vi "Drive Test.vi"   [LabVIEW 2018]
types:
  T1 = cluster{"Reverse (T) / Normal (F)":bool, "Power Scaling (1=Normal) ":dbl, "Deadband Value":dbl}
  T2 = typedef "WPI_MotorControlDeviceRef.ctl" = cluster{"DeviceStatus":errorcluster, "Type":T3, "PWM":cluster{"PWM Channel":T4, "DeadBand":T5}, "CAN":cluster{"Device Number":u8, "SetOutput VI Ref":variant, "GetOutput VI Ref":variant, "Enable VI Ref":variant, "Disable VI Ref":variant, "Data":variant}, "Invert":bool, "DIO PWM":cluster{"PWM \"Enable\" Channel":T4, "DIOChannel":T6, "PWM Rate":dbl}}
  T3 = typedef "WPI_MotorControlType.ctl" = enum16{"PWM", "CAN", "DIO PWM"}
  T4 = typedef "FPGA_DIOPWMChannel.ctl" = enum8{"PWM 0", "PWM 1", "PWM 2", "PWM 3", "PWM 4", "PWM 5", "PWM 6", "PWM 7", "PWM 8", "PWM 9", "PWM MXP 0", "PWM MXP 1", "PWM MXP 2", "PWM MXP 3", "PWM MXP 4", "PWM MXP 5", "PWM MXP 6", "PWM MXP 7", "PWM MXP 8", "PWM MXP 9", "Invalid"}
  T5 = typedef "WPI_PWMDeadband.ctl" = cluster{"Name":string, "maxPositivePwm":i32, "minPositivePwm":i32, "centerPwm":i32, "maxNegativePwm":i32, "minNegativePwm":i32, "angularRange":u16}
  T6 = typedef "FPGA_DIOChannel.ctl" = enum8{"DIO 0", "DIO 1", "DIO 2", "DIO 3", "DIO 4", "DIO 5", "DIO 6", "DIO 7", "DIO 8", "DIO 9", "DIO MXP 0", "DIO MXP 1", "DIO MXP 2", "DIO MXP 3", "DIO MXP 4", "DIO MXP 5", "DIO MXP 6", "DIO MXP 7", "DIO MXP 8", "DIO MXP 9", "DIO MXP 10", "DIO MXP 11", "DIO MXP 12", "DIO MXP 13", "DIO MXP 14", "DIO MXP 15", "SPI Port CS1", "SPI Port CS2", "SPI Port CS3", "SPI Port MISO", "SPI Port MOSI", "Invalid"}
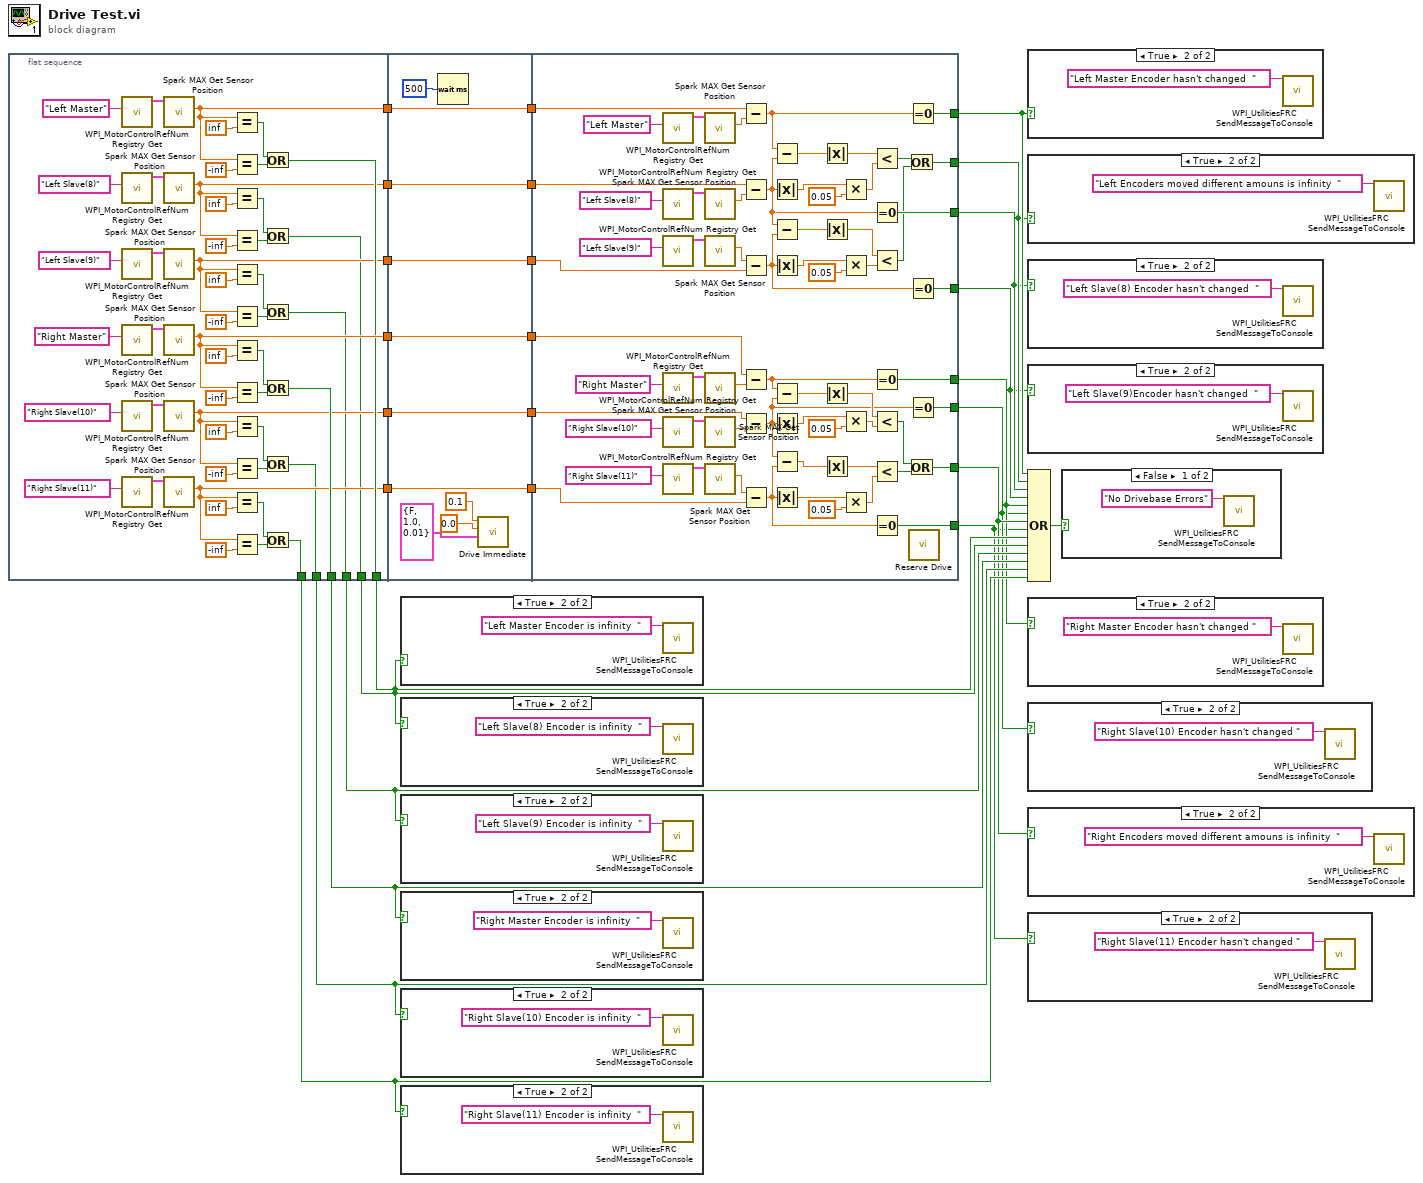
[diagram p0: block diagram]
diagram:
  n1 = flat-sequence {
    tunnel: [w63] -> w27
    tunnel: [w62] -> w26
    tunnel: [w61] -> w14
    tunnel: [w60] -> w11
    tunnel: [w47] -> w22
    tunnel: [w46] -> w20
    tunnel: [w44] -> w17
    tunnel: [w45] -> w16
    tunnel: [w31] -> w13
    tunnel: [w30] -> w12
    tunnel: [w29] -> w10
    tunnel: [w28] -> w9
    tunnel: w27 -> [w82]
    tunnel: [w82] -> w25
    tunnel: w26 -> [w81]
    tunnel: [w81] -> w24
    tunnel: [w79] -> w23
    tunnel: w22 -> [w79]
    tunnel: [w78] -> w21
    tunnel: w20 -> [w78]
    tunnel: [w76] -> w19
    tunnel: [w77] -> w18
    tunnel: w17 -> [w76]
    tunnel: w16 -> [w77]
    tunnel: w25 -> [w143]
    tunnel: w24 -> [w128]
    tunnel: [w133] -> w8
    tunnel: [w126] -> w3
    tunnel: w23 -> [w130]
    tunnel: w21 -> [w90]
    tunnel: w19 -> [w125]
    tunnel: w18 -> [w92]
    tunnel: [w132] -> w6
    tunnel: [w129] -> w4
    tunnel: [w123] -> w2
    tunnel: [w122] -> w1
    tunnel: [w88] -> w7
    tunnel: [w87] -> w5
    frame #0 {
      n2 = call <vilib>:"WPI_MotorControlRefNum Registry Get.vi"("refnum name"="Left Master") -> ("MotorControlDevRef"=w75:T2)  [unwired: 9 in, 1 out]
      n3 = call <vilib>:"WPI_MotorControlRefNum Registry Get.vi"("refnum name"="Left Slave(8)") -> ("MotorControlDevRef"=w49:T2)  [unwired: 9 in, 1 out]
      n4 = call <vilib>:"WPI_MotorControlRefNum Registry Get.vi"("refnum name"="Left Slave(9)") -> ("MotorControlDevRef"=w48:T2)  [unwired: 9 in, 1 out]
      n5 = call <vilib>:"WPI_MotorControlRefNum Registry Get.vi"("refnum name"="Right Master") -> ("MotorControlDevRef"=w74:T2)  [unwired: 9 in, 1 out]
      n6 = call <vilib>:"WPI_MotorControlRefNum Registry Get.vi"("refnum name"="Right Slave(10)") -> ("MotorControlDevRef"=w42:T2)  [unwired: 9 in, 1 out]
      n7 = call <vilib>:"WPI_MotorControlRefNum Registry Get.vi"("refnum name"="Right Slave(11)") -> ("MotorControlDevRef"=w43:T2)  [unwired: 9 in, 1 out]
      n8 = call <vilib>:"Spark MAX Get Sensor Position.vi"("MotorControlDevRef in"=w75) -> ("Sensor Position"=w63:dbl)  [unwired: 7 in, 3 out]
      n9 = call <vilib>:"Spark MAX Get Sensor Position.vi"("MotorControlDevRef in"=w49) -> ("Sensor Position"=w47:dbl)  [unwired: 7 in, 3 out]
      n10 = call <vilib>:"Spark MAX Get Sensor Position.vi"("MotorControlDevRef in"=w48) -> ("Sensor Position"=w46:dbl)  [unwired: 7 in, 3 out]
      n11 = call <vilib>:"Spark MAX Get Sensor Position.vi"("MotorControlDevRef in"=w74) -> ("Sensor Position"=w62:dbl)  [unwired: 7 in, 3 out]
      n12 = call <vilib>:"Spark MAX Get Sensor Position.vi"("MotorControlDevRef in"=w42) -> ("Sensor Position"=w44:dbl)  [unwired: 7 in, 3 out]
      n13 = call <vilib>:"Spark MAX Get Sensor Position.vi"("MotorControlDevRef in"=w43) -> ("Sensor Position"=w45:dbl)  [unwired: 7 in, 3 out]
      n14 = Equal?(x=w63, y=inf) -> (x = y?=w68:bool)
      n15 = Equal?(x=w63, y=-inf) -> (x = y?=w69:bool)
      n16 = Equal?(x=w47, y=inf) -> (x = y?=w56:bool)
      n17 = Equal?(x=w47, y=-inf) -> (x = y?=w57:bool)
      n18 = Equal?(x=w46, y=inf) -> (x = y?=w55:bool)
      n19 = Equal?(x=w46, y=-inf) -> (x = y?=w54:bool)
      n20 = Equal?(x=w62, y=inf) -> (x = y?=w67:bool)
      n21 = Equal?(x=w62, y=-inf) -> (x = y?=w66:bool)
      n22 = Equal?(x=w44, y=inf) -> (x = y?=w35:bool)
      n23 = Equal?(x=w44, y=-inf) -> (x = y?=w34:bool)
      n24 = Equal?(x=w45, y=inf) -> (x = y?=w36:bool)
      n25 = Equal?(x=w45, y=-inf) -> (x = y?=w37:bool)
      n26 = Or(x=w68, y=w69) -> (x .or. y?=w61:bool)
      n27 = Or(x=w56, y=w57) -> (x .or. y?=w31:bool)
      n28 = Or(x=w55, y=w54) -> (x .or. y?=w30:bool)
      n29 = Or(x=w67, y=w66) -> (x .or. y?=w60:bool)
      n30 = Or(x=w35, y=w34) -> (x .or. y?=w29:bool)
      n31 = Or(x=w36, y=w37) -> (x .or. y?=w28:bool)
    }
    frame #1 {
      n32 = Wait (ms)(milliseconds to wait=u32 500) -> ()  [unwired: 1 out]
      n33 = call "Drive Immediate.vi"("Modifiers"=T1 {"Reverse (T) / Normal (F)"=FALSE, "Power Scaling (1=Normal) "=1.0, "Deadband Value"=0.01}, "Right Setpoint (Turning)"=0.0, "Left Setpoint (Power)"=0.1) -> ()  [unwired: 8 in, 1 out]
    }
    frame #2 {
      n34 = call <vilib>:"WPI_MotorControlRefNum Registry Get.vi"("refnum name"="Left Master") -> ("MotorControlDevRef"=w144:T2)  [unwired: 9 in, 1 out]
      n35 = call <vilib>:"WPI_MotorControlRefNum Registry Get.vi"("refnum name"="Left Slave(8)") -> ("MotorControlDevRef"=w140:T2)  [unwired: 9 in, 1 out]
      n36 = call <vilib>:"WPI_MotorControlRefNum Registry Get.vi"("refnum name"="Left Slave(9)") -> ("MotorControlDevRef"=w141:T2)  [unwired: 9 in, 1 out]
      n37 = call <vilib>:"WPI_MotorControlRefNum Registry Get.vi"("refnum name"="Right Master") -> ("MotorControlDevRef"=w145:T2)  [unwired: 9 in, 1 out]
      n38 = call <vilib>:"WPI_MotorControlRefNum Registry Get.vi"("refnum name"="Right Slave(10)") -> ("MotorControlDevRef"=w135:T2)  [unwired: 9 in, 1 out]
      n39 = call <vilib>:"WPI_MotorControlRefNum Registry Get.vi"("refnum name"="Right Slave(11)") -> ("MotorControlDevRef"=w134:T2)  [unwired: 9 in, 1 out]
      n40 = call <vilib>:"Spark MAX Get Sensor Position.vi"("MotorControlDevRef in"=w144) -> ("Sensor Position"=w142:dbl)  [unwired: 7 in, 3 out]
      n41 = call <vilib>:"Spark MAX Get Sensor Position.vi"("MotorControlDevRef in"=w140) -> ("Sensor Position"=w131:dbl)  [unwired: 7 in, 3 out]
      n42 = call <vilib>:"Spark MAX Get Sensor Position.vi"("MotorControlDevRef in"=w141) -> ("Sensor Position"=w91:dbl)  [unwired: 7 in, 3 out]
      n43 = call <vilib>:"Spark MAX Get Sensor Position.vi"("MotorControlDevRef in"=w145) -> ("Sensor Position"=w127:dbl)  [unwired: 7 in, 3 out]
      n44 = call <vilib>:"Spark MAX Get Sensor Position.vi"("MotorControlDevRef in"=w135) -> ("Sensor Position"=w124:dbl)  [unwired: 7 in, 3 out]
      n45 = call <vilib>:"Spark MAX Get Sensor Position.vi"("MotorControlDevRef in"=w134) -> ("Sensor Position"=w89:dbl)  [unwired: 7 in, 3 out]
      n46 = Subtract(x=w143, y=w142) -> (x-y=w121:dbl)
      n47 = Subtract(x=w130, y=w131) -> (x-y=w110:dbl)
      n48 = Subtract(x=w91, y=w90) -> (x-y=w109:dbl)
      n49 = Subtract(x=w128, y=w127) -> (x-y=w97:dbl)
      n50 = Subtract(x=w125, y=w124) -> (x-y=w98:dbl)
      n51 = Subtract(x=w89, y=w92) -> (x-y=w86:dbl)
      n52 = Subtract(x=w121, y=w110) -> (x-y=w120:dbl)
      n53 = Absolute Value(x=w110) -> (abs(x)=w118:dbl)
      n54 = Subtract(x=w110, y=w109) -> (x-y=w111:dbl)
      n55 = Absolute Value(x=w109) -> (abs(x)=w113:dbl)
      n56 = Subtract(x=w97, y=w98) -> (x-y=w99:dbl)
      n57 = Absolute Value(x=w98) -> (abs(x)=w101:dbl)
      n58 = Subtract(x=w98, y=w86) -> (x-y=w108:dbl)
      n59 = Absolute Value(x=w86) -> (abs(x)=w106:dbl)
      n60 = Absolute Value(x=w120) -> (abs(x)=w119:dbl)
      n61 = Absolute Value(x=w111) -> (abs(x)=w112:dbl)
      n62 = Absolute Value(x=w99) -> (abs(x)=w100:dbl)
      n63 = Absolute Value(x=w108) -> (abs(x)=w107:dbl)
      n64 = Multiply(x=w118, y=0.05) -> (x*y=w116:dbl)
      n65 = Multiply(x=w113, y=0.05) -> (x*y=w115:dbl)
      n66 = Multiply(x=w101, y=0.05) -> (x*y=w103:dbl)
      n67 = Multiply(x=w106, y=0.05) -> (x*y=w104:dbl)
      n68 = Less?(x=w119, y=w116) -> (x < y?=w96:bool)
      n69 = Equal To 0?(x=w110) -> (x = 0?=w132:bool)
      n70 = Less?(x=w112, y=w115) -> (x < y?=w95:bool)
      n71 = Equal To 0?(x=w97) -> (x = 0?=w126:bool)
      n72 = Less?(x=w100, y=w103) -> (x < y?=w94:bool)
      n73 = Less?(x=w107, y=w104) -> (x < y?=w93:bool)
      n74 = Equal To 0?(x=w86) -> (x = 0?=w122:bool)
      n75 = Or(x=w96, y=w95) -> (x .or. y?=w88:bool)
      n76 = Or(x=w94, y=w93) -> (x .or. y?=w87:bool)
      n77 = Equal To 0?(x=w121) -> (x = 0?=w133:bool)
      n78 = Equal To 0?(x=w109) -> (x = 0?=w129:bool)
      n79 = Equal To 0?(x=w98) -> (x = 0?=w123:bool)
      n80 = call "Reserve Drive.vi"() -> ()  [unwired: 11 in, 1 out]
    }
  }
  n81 = case shown="True" w14 {
    frame False {
    }
    frame True {
      n82 = call <vilib>:"WPI_UtilitiesFRC SendMessageToConsole.vi"("Message"="Left Master Encoder is infinity  " ("t")) -> ()  [unwired: 14 in, 1 out]
    }
  }
  n83 = case shown="True" w13 {
    frame False {
    }
    frame True {
      n84 = call <vilib>:"WPI_UtilitiesFRC SendMessageToConsole.vi"("Message"="Left Slave(8) Encoder is infinity  " ("t")) -> ()  [unwired: 14 in, 1 out]
    }
  }
  n85 = case shown="True" w12 {
    frame False {
    }
    frame True {
      n86 = call <vilib>:"WPI_UtilitiesFRC SendMessageToConsole.vi"("Message"="Left Slave(9) Encoder is infinity  " ("t")) -> ()  [unwired: 14 in, 1 out]
    }
  }
  n87 = case shown="True" w11 {
    frame False {
    }
    frame True {
      n88 = call <vilib>:"WPI_UtilitiesFRC SendMessageToConsole.vi"("Message"="Right Master Encoder is infinity  " ("t")) -> ()  [unwired: 14 in, 1 out]
    }
  }
  n89 = case shown="True" w10 {
    frame False {
    }
    frame True {
      n90 = call <vilib>:"WPI_UtilitiesFRC SendMessageToConsole.vi"("Message"="Right Slave(10) Encoder is infinity  " ("t")) -> ()  [unwired: 14 in, 1 out]
    }
  }
  n91 = case shown="True" w9 {
    frame False {
    }
    frame True {
      n92 = call <vilib>:"WPI_UtilitiesFRC SendMessageToConsole.vi"("Message"="Right Slave(11) Encoder is infinity  " ("t")) -> ()  [unwired: 14 in, 1 out]
    }
  }
  n93 = case shown="True" w8 {
    frame False {
    }
    frame True {
      n94 = call <vilib>:"WPI_UtilitiesFRC SendMessageToConsole.vi"("Message"="Left Master Encoder hasn't changed  " ("t")) -> ()  [unwired: 14 in, 1 out]
    }
  }
  n95 = case shown="True" w7 {
    frame False {
    }
    frame True {
      n96 = call <vilib>:"WPI_UtilitiesFRC SendMessageToConsole.vi"("Message"="Left Encoders moved different amouns is infinity  " ("t")) -> ()  [unwired: 14 in, 1 out]
    }
  }
  n97 = case shown="True" w6 {
    frame False {
    }
    frame True {
      n98 = call <vilib>:"WPI_UtilitiesFRC SendMessageToConsole.vi"("Message"="Left Slave(8) Encoder hasn't changed  " ("t")) -> ()  [unwired: 14 in, 1 out]
    }
  }
  n99 = case shown="True" w4 {
    frame False {
    }
    frame True {
      n100 = call <vilib>:"WPI_UtilitiesFRC SendMessageToConsole.vi"("Message"="Left Slave(9)Encoder hasn't changed  " ("t")) -> ()  [unwired: 14 in, 1 out]
    }
  }
  n101 = Compound Arithmetic op=OR(w8, w7, w6, w4, w3, w2, w5, w1, w14, w13, w12, w11, w10, w9) -> (w15:bool)
  n102 = case shown="True" w3 {
    frame False {
    }
    frame True {
      n103 = call <vilib>:"WPI_UtilitiesFRC SendMessageToConsole.vi"("Message"="Right Master Encoder hasn't changed " ("t")) -> ()  [unwired: 14 in, 1 out]
    }
  }
  n104 = case shown="True" w2 {
    frame False {
    }
    frame True {
      n105 = call <vilib>:"WPI_UtilitiesFRC SendMessageToConsole.vi"("Message"="Right Slave(10) Encoder hasn't changed " ("t")) -> ()  [unwired: 14 in, 1 out]
    }
  }
  n106 = case shown="True" w5 {
    frame False {
    }
    frame True {
      n107 = call <vilib>:"WPI_UtilitiesFRC SendMessageToConsole.vi"("Message"="Right Encoders moved different amouns is infinity  " ("t")) -> ()  [unwired: 14 in, 1 out]
    }
  }
  n108 = case shown="True" w1 {
    frame False {
    }
    frame True {
      n109 = call <vilib>:"WPI_UtilitiesFRC SendMessageToConsole.vi"("Message"="Right Slave(11) Encoder hasn't changed " ("t")) -> ()  [unwired: 14 in, 1 out]
    }
  }
  n110 = case shown="False" w15 {
    frame False {
      n111 = call <vilib>:"WPI_UtilitiesFRC SendMessageToConsole.vi"("Message"="No Drivebase Errors" ("f")) -> ()  [unwired: 14 in, 1 out]
    }
    frame True {
    }
  }
